vi "BkgGradient.vi"(11 "General settings":T1) -> (0 "Holo mask":dbl[][](array[numeric]), 3 "gradient":dbl[][](array[numeric]))   [LabVIEW 2014]
uses:
  Controls/SLM General Settings.ctl
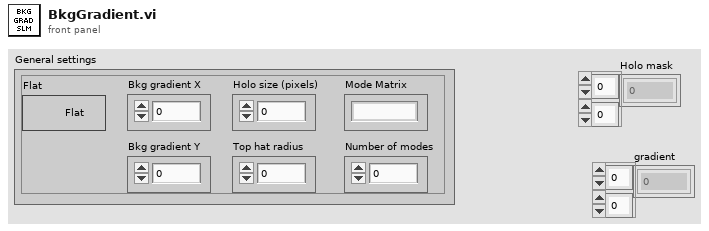
[diagram p1: front panel]
types:
  T1 = typedef "SLM General Settings.ctl" = cluster{"Holo size (pixels)":i32, "Top hat radius":dbl, "Number of modes":i32, "Bkg gradient X":dbl, "Bkg gradient Y":dbl, "Flat":bool, "Mode Matrix":u16}
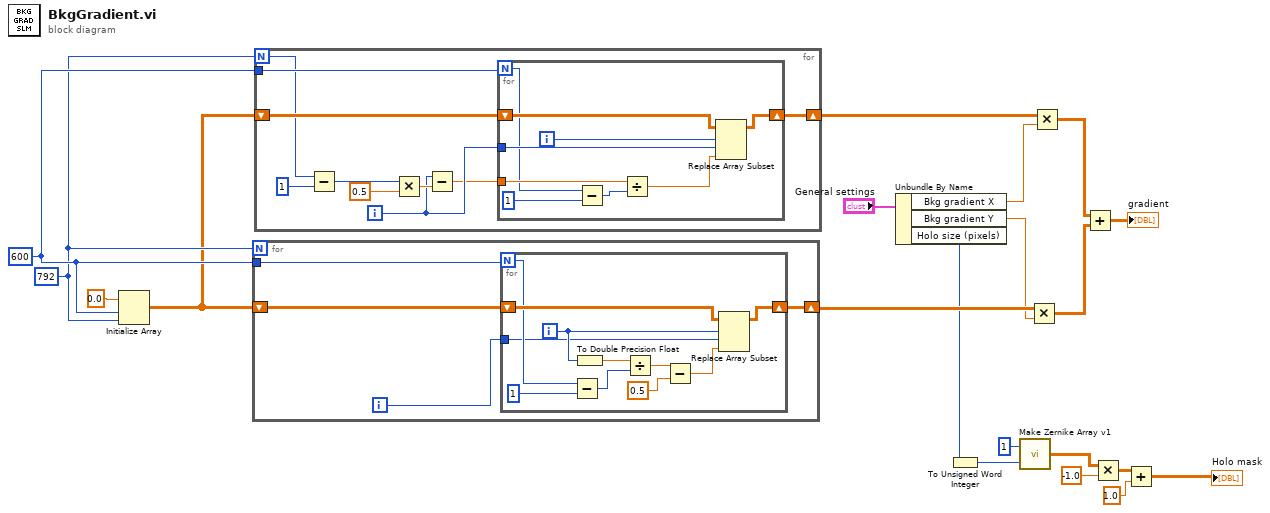
[diagram p0: block diagram]
diagram:
  w19 = 792 ("dimension size")
  w20 = 600
  n1 = Initialize Array(0.0 ("element"), w20, w19) -> (w18:dbl[][])
  n2 = for {
    N: w19 -> [_]
    tunnel: w20 -> [w23]
    shift-right: [w22] -> w9
    shift-left: w18 -> [w24]
    i -> [w21]
    n3 = for {
      N: w23 -> [w27]
      shift-right: [w34] -> w22
      shift-left: w24 -> [w33]
      tunnel: w21 -> [w25]
      i -> [w35]
      n4 = Subtract(x=w27, y=1) -> (x-y=w28:i32)
      n5 = To Double Precision Float(number=w35) -> (double precision float=w32:dbl)
      n6 = Divide(x=w32, y=w28) -> (x/y=w30:dbl)
      n7 = Subtract(x=w30, y=0.5 ("element")) -> (x-y=w29:dbl)
      n8 = Replace Array Subset(array=w33, new element=w29, index (row)=w35, index (col)=w25) -> (w34:dbl[][])
    }
  }
  n9 = for {
    N: w19 -> [w38]
    tunnel: w20 -> [w44]
    shift-right: [w43] -> w10
    shift-left: w18 -> [w45]
    i -> [w40]
    n10 = Subtract(x=w38, y=1) -> (x-y=w37:i32)
    n11 = Multiply(x=w37, y=0.5 ("element")) -> (x*y=w41:dbl)
    n12 = Subtract(x=w40, y=w41) -> (x-y=w39:dbl)
    n13 = for {
      N: w44 -> [w47]
      shift-right: [w53] -> w43
      shift-left: w45 -> [w52]
      tunnel: w40 -> [w51]
      tunnel: w39 -> [w50]
      i -> [w54]
      n14 = Subtract(x=w47, y=1) -> (x-y=w46:i32)
      n15 = Divide(x=w50, y=w46) -> (x/y=w49:dbl)
      n16 = Replace Array Subset(array=w52, new element=w49, index (row)=w54, index (col)=w51) -> (w53:dbl[][])
    }
  }
  n17 = Unbundle By Name("General settings") -> ("Bkg gradient X"=w4:dbl, "Bkg gradient Y"=w3:dbl, "Holo size (pixels)"=w2:i32)
  n18 = To Unsigned Word Integer(number=w2) -> (unsigned 16bit integer=w1:u16)
  n19 = call "Make Zernike Array v1.vi"("size"=w1, "z"=u8 1) -> ("zernike array"=w14:dbl[][])
  n20 = Multiply(x=w9, y=w3) -> (x*y=w7:dbl[][])
  n21 = Multiply(x=w10, y=w4) -> (x*y=w8:dbl[][])
  n22 = Add(x=w8, y=w7) -> (x+y=→"gradient":dbl[][])
  n23 = Multiply(x=w14, y=-1.0) -> (x*y=w13:dbl[][])
  n24 = Add(x=w13, y=1.0) -> (x+y=→"Holo mask":dbl[][])
